vi "KINECT_Index.vi"(8 "Arm Drive Min in (Reverse)":dbl, 9 "Arm Drive Max in (Forward)":dbl, 10 "Z Wrist Left":dbl, 11 "Z Wrist Right":dbl) -> (0 "Z Wrist Left":sgl, 1 "Z Wrist Right":sgl, 3 "Kinect Command":string, 4 "Arm Drive Min out (Reverse)":dbl, 5 "Arm Drive Max out (Forward)":dbl)   [LabVIEW 2012]
uses:
  <vilib>/addons/Kinect/Skeleton Vertex Index.ctl
panel:
  out "Go to Calibrate":bool
  in  "Muscle Tolerance":dbl=0.05
  out "In The Middle ?":bool
  out "?":dbl(slide) scale=2.4213576316833496..2.7618839740753174
  out "Current Max":dbl
  out "Current Min":dbl
  out "Average Current Position (Both Hands)":dbl
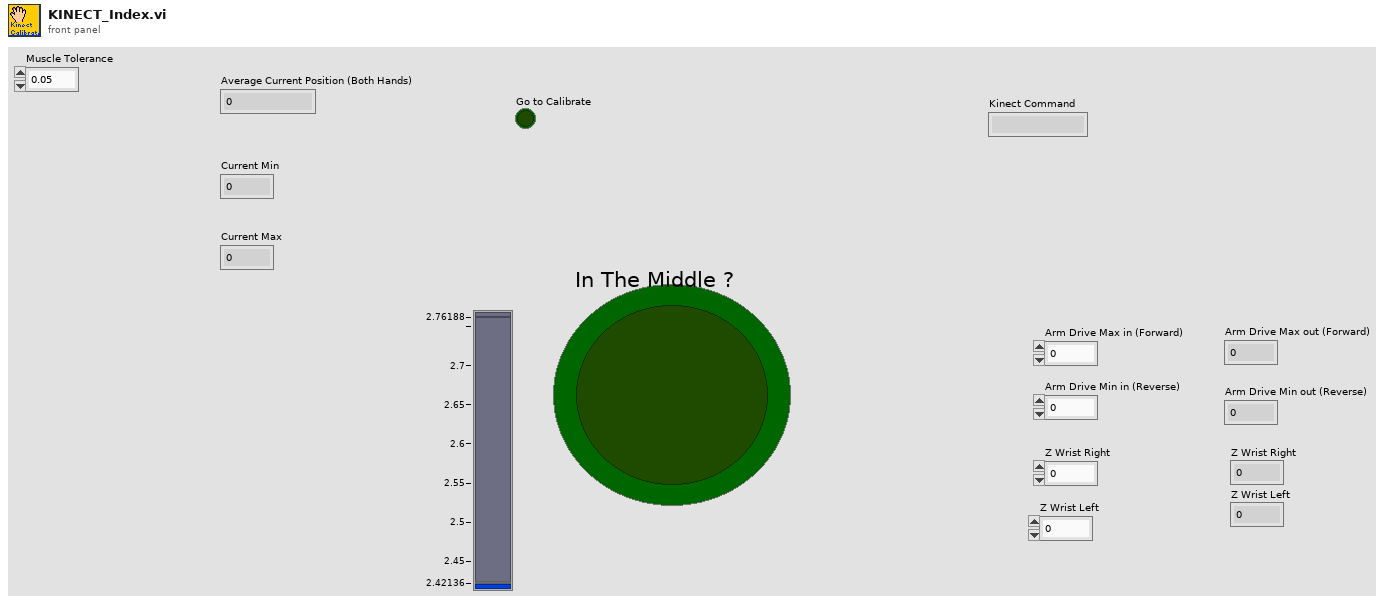
[diagram p1: front panel]
types:
  T1 = typedef "Skeleton Vertex Index.ctl" = i32
  T2 = enum16{"Enable", "Set/Reset", "Run Timer", "Read/Store"}
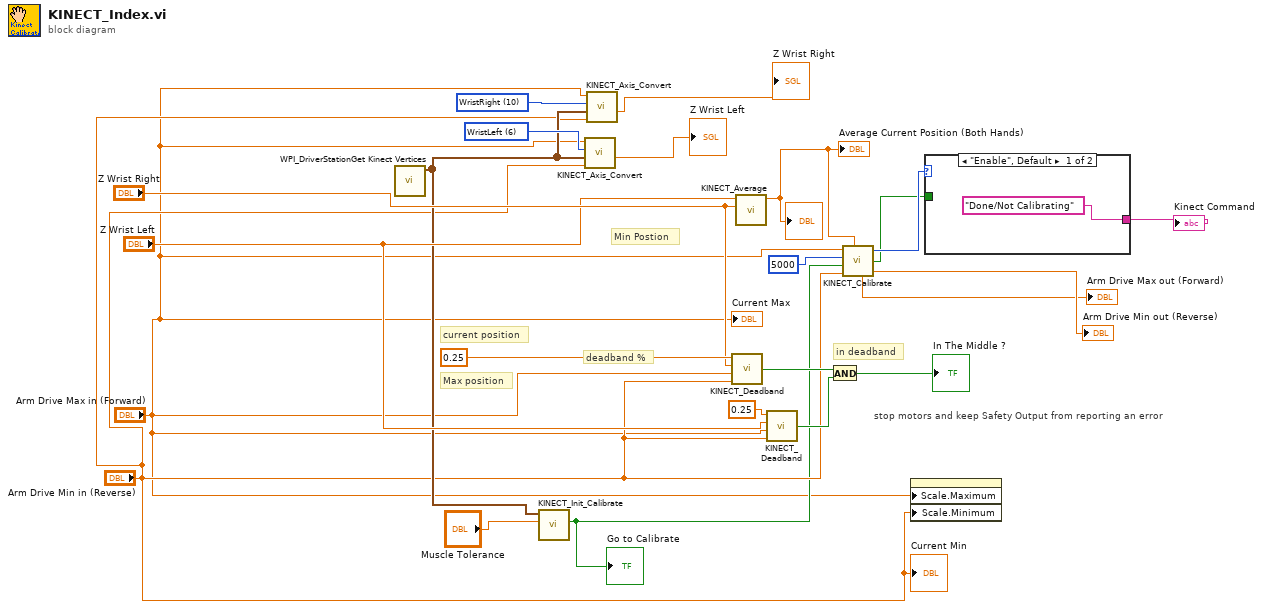
[diagram p0: block diagram]
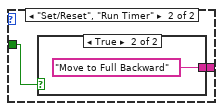
[diagram p2: hidden frame]
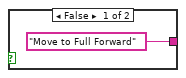
[diagram p3: hidden frame]
diagram:
  w22 = T1 10 items=["HipCenter", "Spine", "ShoulderCenter", "Head", "ShoulderLeft", "ElbowLeft", "WristLeft", "HandLeft", "ShoulderRight", "ElbowRight", "WristRight", "HandRight", "HipLeft", "KneeLeft", "AnkleLeft", "FootLeft", "HipRight", "KneeRight", "AnkleRight", "FootRight"] ("Skeleton Joints")
  w23 = T1 6 items=["HipCenter", "Spine", "ShoulderCenter", "Head", "ShoulderLeft", "ElbowLeft", "WristLeft", "HandLeft", "ShoulderRight", "ElbowRight", "WristRight", "HandRight", "HipLeft", "KneeLeft", "AnkleLeft", "FootLeft", "HipRight", "KneeRight", "AnkleRight", "FootRight"] ("Skeleton Joints")
  # "deadband %"
  # "Min Postion"
  # "Max position"
  # "current position"
  # "in deadband"
  # "stop motors and keep Safety Output from reporting an error"
  n1 = call <vilib>:"WPI_DriverStationGet Kinect Vertices.vi"() -> ("Skeleton Vertices"=w11:cluster{"x":sgl, "y":sgl, "z":sgl}[])  [unwired: 10 in, 1 out]
  n2 = call "KINECT_Init_Calibrate.vi"("Muscle Tolerance"="Muscle Tolerance", "Skeleton Vertices"=w11) -> ("Go to Calibrate"=w4:bool)  [unwired: 9 in]
  "Go to Calibrate" <- w4
  n3 = call "KINECT_Axis_Convert.vi"("Arm Drive Min (Reverse)"="Arm Drive Min in (Reverse)", "Skeleton Vertices"=w11, "Wrist Input"=w23, "Arm Drive Max (Forward)"="Arm Drive Max in (Forward)") -> ("Z Axis Out"=→"Z Wrist Left":sgl)  [unwired: 5 in, 2 out]
  n4 = call "KINECT_Axis_Convert.vi"("Arm Drive Min (Reverse)"="Arm Drive Min in (Reverse)", "Skeleton Vertices"=w11, "Wrist Input"=w22, "Arm Drive Max (Forward)"="Arm Drive Max in (Forward)") -> ("Z Axis Out"=→"Z Wrist Right":sgl)  [unwired: 5 in, 2 out]
  n5 = call "KINECT_Deadband.vi"("Min"="Arm Drive Min in (Reverse)", "Max"="Arm Drive Max in (Forward)", "Current Position"="Z Wrist Right", "Deadband %"=0.25 ("x")) -> ("In Range?"=w20:bool)
  n6 = call "KINECT_Average.vi"("Min"="Z Wrist Right", "Max"="Z Wrist Left") -> ("Average"=w1:dbl)  [unwired: 8 in, 1 out]
  "Average Current Position (Both Hands)" <- w1
  "?" <- w1
  n7 = call "KINECT_Deadband.vi"("Min"="Arm Drive Min in (Reverse)", "Max"="Arm Drive Max in (Forward)", "Current Position"="Z Wrist Left", "Deadband %"=0.25 ("x")) -> ("In Range?"=w18:bool)
  n8 = And(x=w20, y=w18) -> (x .and. y?=→"In The Middle ?":bool)
  n9 = call "KINECT_Calibrate.vi"("Arm Drive Min in (Reverse)"="Arm Drive Min in (Reverse)", "Enable Calibration"=w4, "Current Value"=w1, "Wait Time (ms)"=u32 5000, "Arm Drive Max in (Forward)"="Arm Drive Max in (Forward)") -> ("Arm Drive Min out (Reverse)"=→"Arm Drive Min out (Reverse)":dbl, "Arm Drive Max out (Forward)"=→"Arm Drive Max out (Forward)":dbl, "Calibrating"=w7:bool, "Result"=w8:T2)  [unwired: 2 in]
  n10 = property class="Slide (strict)"("Scale.Maximum"="Arm Drive Max in (Forward)", "Scale.Minimum"="Arm Drive Min in (Reverse)") -> ()  [unwired: 2 in, 2 out]
  n11 = case shown="\"Enable\", Default" w8 {
    tunnel: w7 -> [_ w26]
    tunnel: ["Done/Not Calibrating" w25] -> w10
    frame "Enable", Default {
    }
    frame "Set/Reset", "Run Timer" {
      n12 = case shown="True" w26 {
        tunnel: ["Move to Full Forward" "Move to Full Backward"] -> w25
        frame False {
        }
        frame True {
        }
      }
    }
  }
  "Kinect Command" <- w10
  "Current Min" <- "Arm Drive Min in (Reverse)"
  "Current Max" <- "Arm Drive Max in (Forward)"
